vi "señal_sensores.vi"() -> ()   [LabVIEW 2018]
uses:
  <vilib>/Utility/file.llb/Read Delimited Spreadsheet (string).vi
panel:
  in  "Multicolumn Listbox":i32(listbox)
  out "display":string[][](array[string])
  out "pt100":i32
  out "ntc":i32
  out "lm35":i32
  # "lm35"
  # "ntc"
  # "pt100"
  # "fecha"
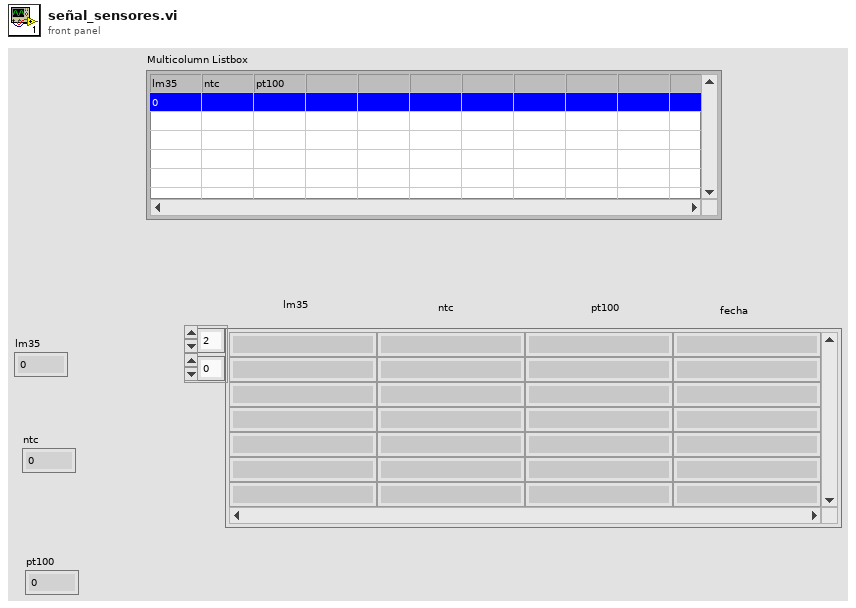
[diagram p1: front panel]
types:
  T1 = enum16{"open", "replace", "create", "open or create", "replace or create", "replace or create with confirmation"}
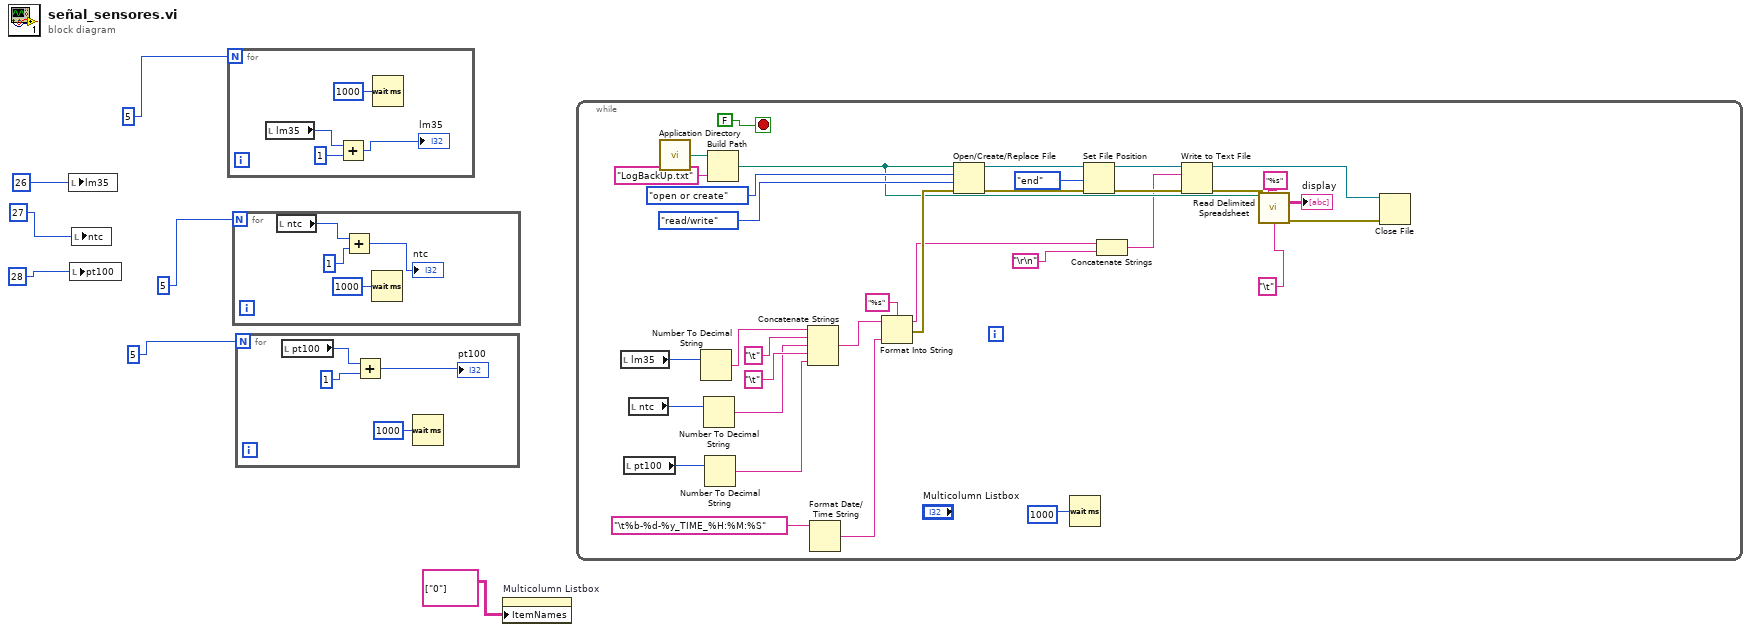
[diagram p0: block diagram]
diagram:
  n1 = local write "lm35"(26 ("Numeric")) -> ()
  n2 = local write "pt100"(28 ("Numeric")) -> ()
  n3 = local write "ntc"(27 ("Numeric")) -> ()
  n4 = for {
    N: 5 -> [_]
    n5 = local read "lm35"() -> (w11:i32)
    n6 = Add(x=w11, y=1) -> (x+y=→"lm35":i32)
    n7 = Wait (ms)(milliseconds to wait=u32 1000) -> ()  [unwired: 1 out]
  }
  n8 = for {
    N: 5 -> [_]
    n9 = local read "ntc"() -> (w15:i32)
    n10 = Add(x=w15, y=1) -> (x+y=→"ntc":i32)
    n11 = Wait (ms)(milliseconds to wait=u32 1000) -> ()  [unwired: 1 out]
  }
  n12 = for {
    N: 5 -> [_]
    n13 = local read "pt100"() -> (w19:i32)
    n14 = Add(x=w19, y=1) -> (x+y=→"pt100":i32)
    n15 = Wait (ms)(milliseconds to wait=u32 1000) -> ()  [unwired: 1 out]
  }
  n16 = property on="Multicolumn Listbox" class="MCListbox (strict)"("ItemNames"=string[][] [["0"]]) -> ()  [unwired: 2 in, 2 out]
  n17 = while {
    stop <- FALSE stop-if-true
    n18 = local read "lm35"() -> (w24:i32)
    n19 = local read "pt100"() -> (w28:i32)
    n20 = local read "ntc"() -> (w23:i32)
    n21 = call <vilib>:"Application Directory.vi"() -> ("Application Directory"=w52:path)
    n22 = Number To Decimal String(number=w24) -> (decimal integer string=w22:string)  [unwired: 1 in]
    n23 = Number To Decimal String(number=w23) -> (decimal integer string=w21:string)  [unwired: 1 in]
    n24 = Number To Decimal String(number=w28) -> (decimal integer string=w20:string)  [unwired: 1 in]
    n25 = Build Path(base path=w52, name or relative path="LogBackUp.txt") -> (appended path=w30:path)
    n26 = Concatenate Strings(w22, "\t" ("format string"), w21, "\t" ("format string"), w20) -> (w25:string)
    n27 = Format Date/Time String(time format string (%c)="\t%b-%d-%y_TIME_%H:%M:%S") -> (date/time string=w34:string)  [unwired: 2 in]
    n28 = Format Into String(format string="%s", initial string=w25, w34) -> (resulting string=w31:string, error out=w33:errorcluster)  [unwired: 1 in]
    n29 = Open/Create/Replace File(file path (use dialog)=w30, error in=w33, operation (0:open)=T1."open or create", access (0:read/write)=enum16{"read/write", "read-only", "write-only"}."read/write") -> (refnum out=w46:refnum<file>, error out=w45:errorcluster)  [unwired: 2 in, 1 out]
    n30 = Wait (ms)(milliseconds to wait=u32 1000) -> ()  [unwired: 1 out]
    n31 = Set File Position(refnum=w46, from (0:start)=enum16{"start", "end", "current"}."end", error in=w45) -> (refnum out=w47:refnum<file>, error out=w44:errorcluster)  [unwired: 1 in]
    n32 = Concatenate Strings(w31, "\r\n") -> (w26:string)
    n33 = Write to Text File(file (use dialog)=w47, text=w26, error in=w44) -> (refnum out=w38:refnum<file>, error out=w40:errorcluster)  [unwired: 1 in, 1 out]
    n34 = call-poly <vilib>:"Read Delimited Spreadsheet.vi"("file path (dialog if empty)"=w30, "format (%s)"="%s", "error in (no error)"=w40, "delimiter (\\t)"="\t" ("delimiter (\\t)")) -> ("all rows"=→"display":string[][], "error out"=w39:errorcluster)  [unwired: 6 in, 4 out]
    n35 = Close File(refnum=w38, error in=w39) -> ()  [unwired: 2 out]
  }
